vi "Configure Channels.vi"(8 "error in":errorcluster, 11 "DAQmx Base Configure Strategy in":refnum<class "DAQmx Base Configure Strategy.lvclass">) -> (0 "error out":errorcluster, 3 "DAQmx Base Configure Strategy out":refnum<class "DAQmx Base Configure Strategy.lvclass">)   [LabVIEW 2024, in "DAQmx Base Configure Strategy.lvclass"]
uses:
  DAQmx Base Configure Strategy.lvclass
  DAQmx Base Configure Strategy.lvclass/DAQmx Base Configure Strategy.ctl
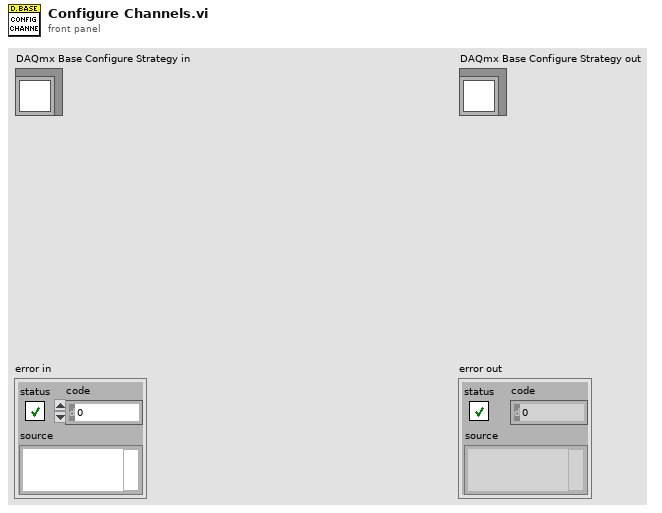
[diagram p1: front panel]
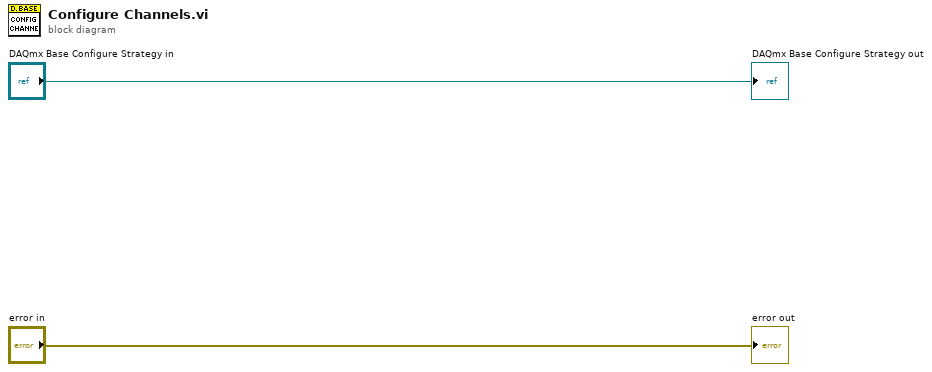
[diagram p0: block diagram]
diagram:
  "error out" <- "error in"
  "DAQmx Base Configure Strategy out" <- "DAQmx Base Configure Strategy in"
